vi "UDPrecieverSucess.vi"() -> ()   [LabVIEW 2012]
panel:
  in  "port":u16=300
  out "Profile":u32[](graph)
  in  "Profile Number":u32=1
  out "Profile Byte by Byte":u8[](graph)
  out "Header Array":bool[][](array[boolean])
  out "NumBins":u32
  out "Cnts/Bin":u32
  out "Prof/Hist":u32
  out "Sync":u32
  out "Channel":u32
  out "rTime":u32
  out "frameCntr":u32
  out "built packet array":string[](array[string])
  out "error post-check":errorcluster
  out "End Reciever Error":errorcluster
  in  "stop reciever":bool
  out "error out post-read":errorcluster
  out "error out pre-read":errorcluster
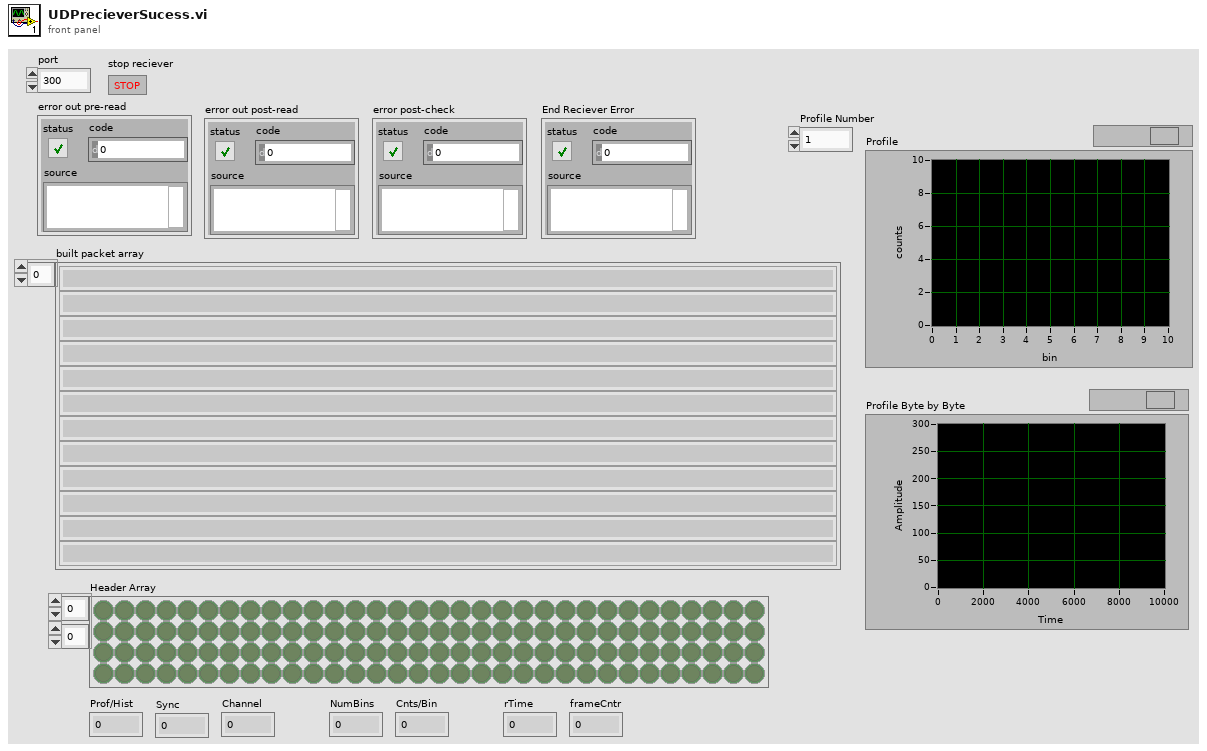
[diagram p1: front panel]
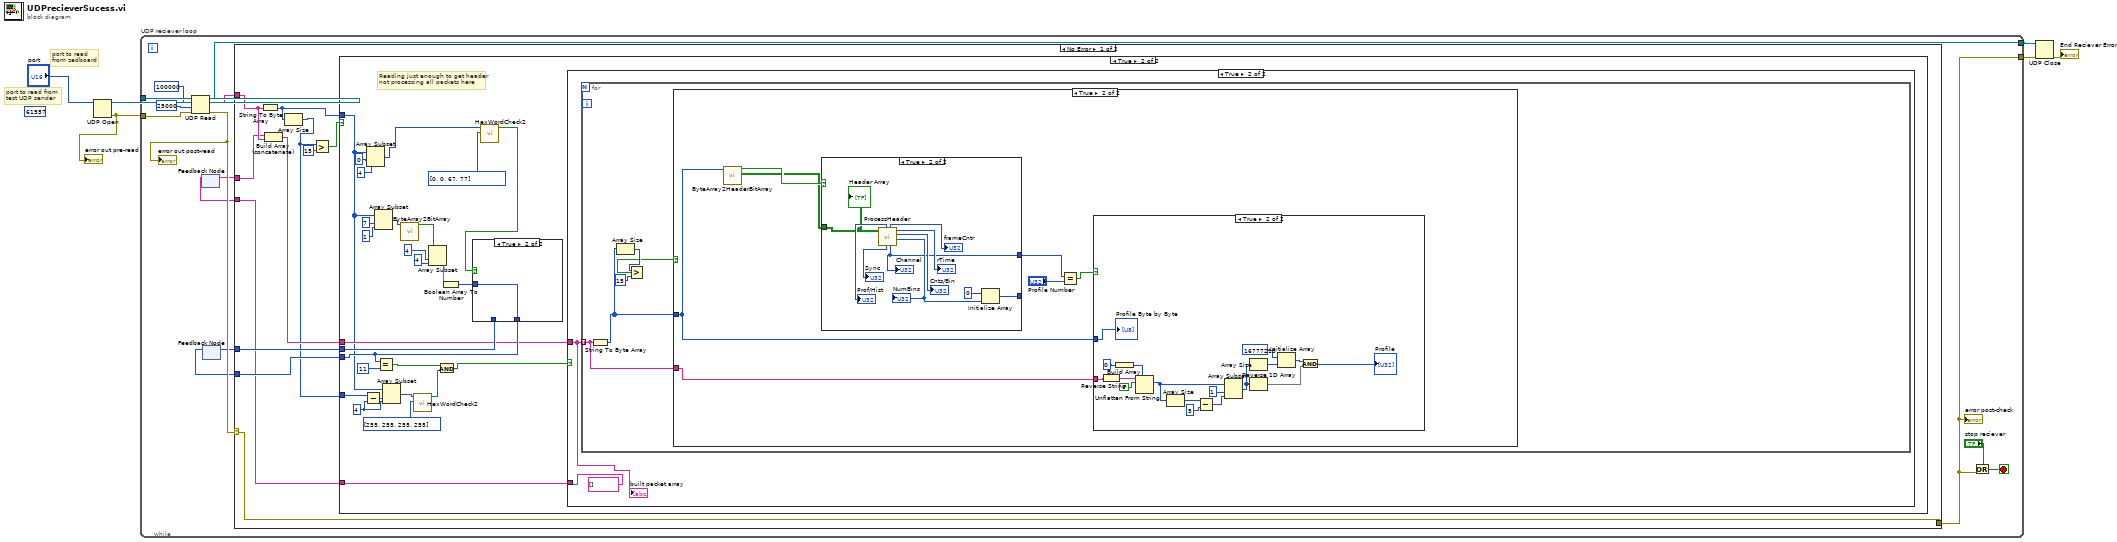
[diagram p0: block diagram]
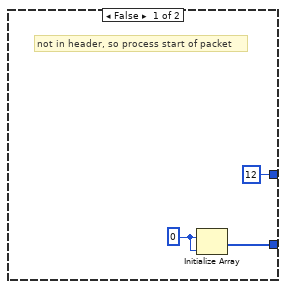
[diagram p6: hidden frame]
diagram:
  (unwired) u16 61557 ("port")
  # "port to read \nfrom zedboard"
  # "port to read from \ntest UDP sender"
  n1 = UDP Open(11:"port") -> (port=w5:refnum<k16>, 0:w2:errorcluster)  [unwired: 4 in, 1 out]
  "error out pre-read" <- w2
  n2 = while "UDP reciever loop" {
    tunnel: [w20] -> w6
    tunnel: w5 -> [w19]
    tunnel: [w12] -> w4
    tunnel: w2 -> [w17]
    stop <- w18 stop-if-true
    n3 = UDP Read(connection ID=w19, max size (548)=100000, timeout ms (25000)=25000, 8:w17) -> (data out=w14:string, error out=w16:errorcluster, 3:w20:refnum<k16>)  [unwired: 2 out]
    "error out post-read" <- w16
    n4 = feedback #1() -> (w9:string[])  [unwired: 1 in]
    n5 = feedback #2() -> (w7:u32)  [unwired: 1 in]
    n6 = case shown="No Error" w16 {
      selector: w16 -> [w31 w110]
      tunnel: w14 -> [w30 _]
      tunnel: [w31 w110] -> w12
      tunnel: [w22 w109] -> w10
      tunnel: w9 -> [w29 w109]
      tunnel: [w26 w108] -> w8
      tunnel: w7 -> [w25 w108]
      frame No Error {
        n7 = String To Byte Array(string=w30) -> (unsigned byte array=w23:u8[])
        n8 = Build Array (concatenate)(w29, w30) -> (w24:string[])
        n9 = Array Size(array=w23) -> (size(s)=w21:i32)
        n10 = Greater?(x=w21, y=15) -> (0:w28:bool)
        n11 = case shown="True" w28 {
          tunnel: w23 -> [_ w43]
          tunnel: [w33 w47] -> w26
          tunnel: w25 -> [w33 w48]
          tunnel: w21 -> [_ w51]
          tunnel: w24 -> [w32 w45]
          tunnel: [w32 w44] -> w22
          frame False {
          }
          frame True {
            w53 = 4 ("length")
            # "Reading just enough to get header\nnot processing all packets here"
            n12 = Subtract(x=w51, y=w53) -> (x-y=w52:i32)
            n13 = Array Subset(array=w43, index=0, length=4) -> (w57:u8[])
            n14 = Array Subset(array=w43, index=7, length=1) -> (w40:u8[])
            n15 = Array Subset(array=w43, index=w52, length=w53) -> (w46:u8[])
            n16 = call "ByteArray2BitArray.vi"("array"=w40) -> ("Array"=w37:bool[])  [unwired: 10 in]
            n17 = call "HexWordCheck2.vi"("array"=u8[] [255, 255, 255, 255], "Input Array"=w46) -> ("Boolean"=w54:bool)  [unwired: 9 in]
            n18 = Array Subset(array=w37, index=4, length=4) -> (w35:bool[])
            n19 = Boolean Array To Number(Boolean array=w35) -> (number=w36:u32)
            n20 = call "HexWordCheck2.vi"("array"=u8[] [0, 0, 67, 77], "Input Array"=w57) -> ("Boolean"=w34:bool)  [unwired: 9 in]
            n21 = case shown="True" w34 {
              tunnel: [w106 w107] -> w47
              tunnel: w48 -> [w106 _]
              tunnel: w36 -> [_ w107]
              frame False {
              }
              frame True {
              }
            }
            n22 = Equal?(x=w47, y=u32 11) -> (x = y?=w50:bool)
            n23 = And(x=w50, y=w54) -> (x .and. y?=w55:bool)
            n24 = case shown="True" w55 {
              tunnel: w45 -> [w61 w62]
              tunnel: [w61 string[] []] -> w44
              frame False {
              }
              frame True {
                n25 = for {
                  tunnel: w62 -> [w64] mode=indexing
                  n26 = String To Byte Array(string=w64) -> (unsigned byte array=w68:u8[])
                  n27 = Array Size(array=w68) -> (size(s)=w67:i32)
                  n28 = Greater?(x=w67, y=15) -> (0:w65:bool)
                  n29 = case shown="True" w65 {
                    tunnel: w68 -> [_ w71]
                    tunnel: w64 -> [_ w70]
                    frame False {
                    }
                    frame True {
                      n30 = call "ByteArray2HeaderBitArray.vi"("Input Byte Array"=w71) -> ("Header Array"=w74:bool[][], "Found Header"=w75:bool)  [unwired: 9 in]
                      n31 = case shown="True" w75 {
                        tunnel: w74 -> [_ w99]
                        tunnel: [w95 w96] -> _
                        tunnel: [u32 12 ("Numeric 4") w97] -> w73
                        frame False {
                          w93 = u32 0 ("element")
                          # "not in header, so process start of packet"
                          n32 = Initialize Array(w93, w93) -> (w95:u32[])
                        }
                        frame True {
                          n33 = call "ProcessHeader.vi"("Array"=w99) -> ("Number of Bins"=w100:u32, "Counts Per Bin"=→"Cnts/Bin":u32, "rTime"=→"rTime":u32, "Channel"=w97:u32, "Frame Counter"=→"frameCntr":u32, "Sync"=→"Sync":u32, "Profiles Per Hist"=→"Prof/Hist":u32)  [unwired: 4 in]
                          "NumBins" <- w100
                          "Channel" <- w97
                          n34 = Initialize Array(u32 0 ("element"), w100) -> (w96:u32[])
                          "Header Array" <- w99
                        }
                      }
                      n35 = Equal?(x=w73, y="Profile Number") -> (x = y?=w72:bool)
                      n36 = case shown="True" w72 {
                        tunnel: w71 -> [_ w92]
                        tunnel: w70 -> [_ w83]
                        frame False {
                        }
                        frame True {
                          n37 = Reverse String(1:w83) -> (0:w82:string)
                          n38 = Build Array(u32 0) -> (w90:u32[])
                          n39 = Unflatten From String(type=w90, binary string=w82, data includes array or string size? (T)=FALSE) -> (value=w88:u32[])  [unwired: 2 in, 2 out]
                          n40 = Array Size(array=w88) -> (size(s)=w87:i32)
                          n41 = Subtract(x=w87, y=5) -> (x-y=w84:i32)
                          n42 = Array Subset(array=w88, index=1, length=w84) -> (w81:u32[])
                          n43 = Reverse 1D Array(array=w81) -> (reversed array=w80:u32[])
                          n44 = Array Size(array=w81) -> (size(s)=w78:i32)
                          n45 = Initialize Array(u32 16777215 ("x*2^n"), w78) -> (w79:u32[])
                          n46 = And(x=w79, y=w80) -> (x .and. y?=→"Profile":u32[])
                          "Profile Byte by Byte" <- w92
                        }
                      }
                    }
                  }
                }
                "built packet array" <- w62
              }
            }
          }
        }
      }
      frame Error {
      }
    }
    "error post-check" <- w12
    n47 = feedback-in #1(w10) -> ()
    n48 = feedback-in #2(w8) -> ()
    n49 = Or(x="stop reciever", y=w12) -> (x .or. y?=w18:bool)
  }
  n50 = UDP Close(connection ID=w6, 8:w4) -> (error out=→"End Reciever Error":errorcluster)  [unwired: 1 out]
